vi "Servo MSMT get DPD Config.vi"(8 "error in (no error)":errorcluster, 11 "Servo MSMT in":refnum<class "Servo MSMT.lvclass">) -> (0 "error out":errorcluster, 1 "USE LUT?":bool, 2 "DPD Enabled?":bool, 3 "Servo MSMT out":refnum<class "Servo MSMT.lvclass">, 4 "LUT":string)   [LabVIEW 2018, in "Servo MSMT.lvlib" / "Servo MSMT.lvclass"]
uses:
  Servo MSMT.lvclass
  Plugins/String Database.lvlibp/String Database.lvclass
  Plugins/Test Group Manager.lvlibp/Test Group Manager.lvclass
  Plugins/Test Group Manager.lvlibp/Includes/Test Group/Test Group.lvclass
  <vilib>/ErrorRing/Error Ring.xnode
  <vilib>/Utility/error.llb/Error Cluster From Error Code.vi
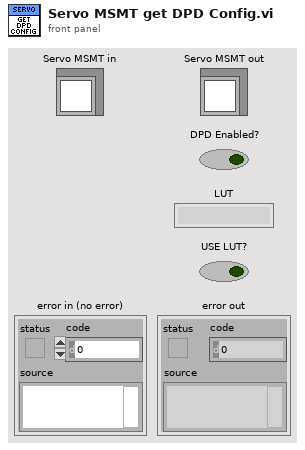
[diagram p1: front panel]
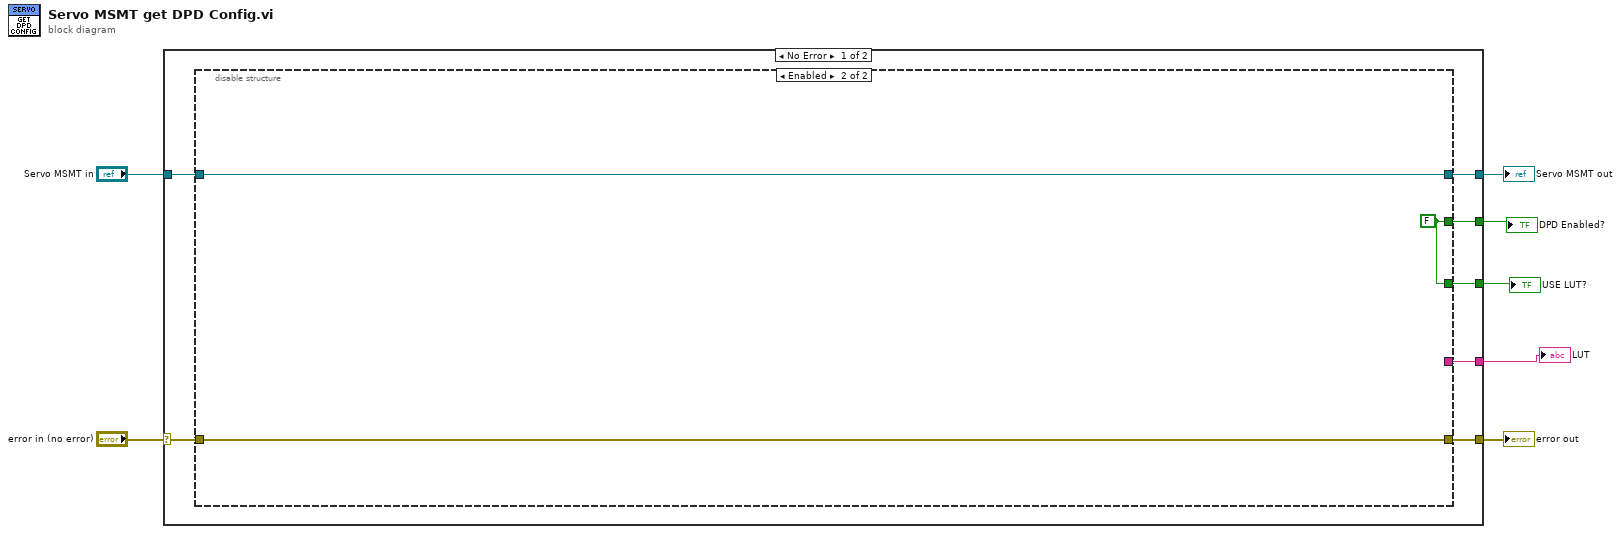
[diagram p0: block diagram]
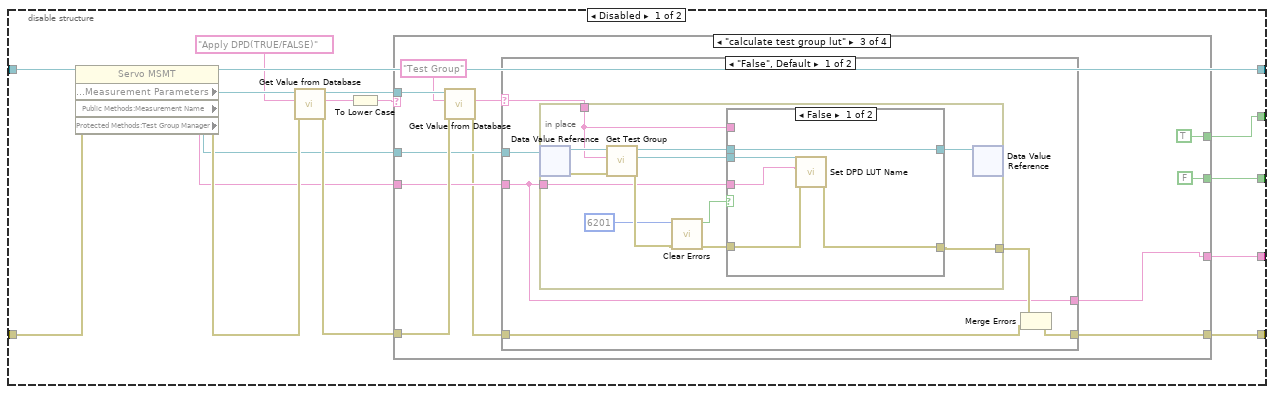
[diagram p2: hidden frame]
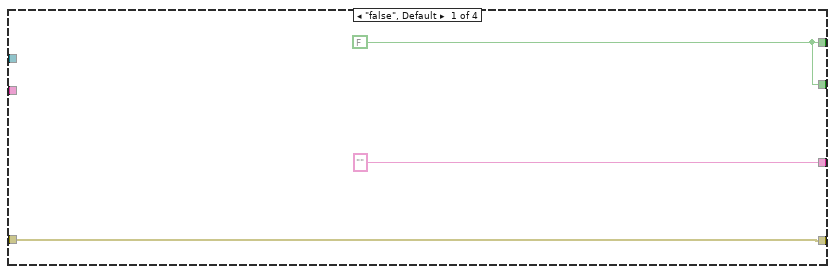
[diagram p3: hidden frame]
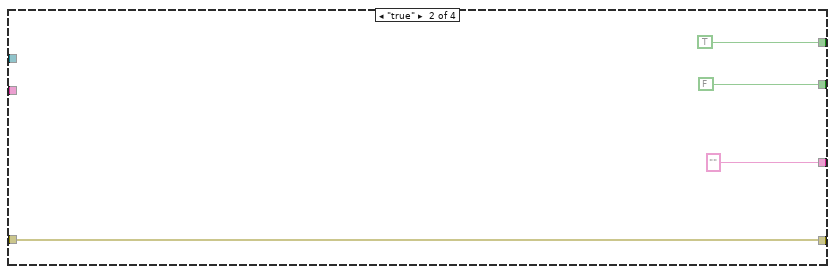
[diagram p4: hidden frame]
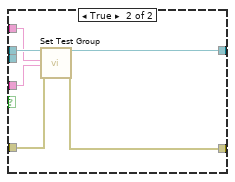
[diagram p5: hidden frame]
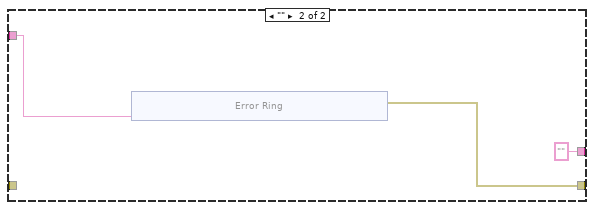
[diagram p6: hidden frame]
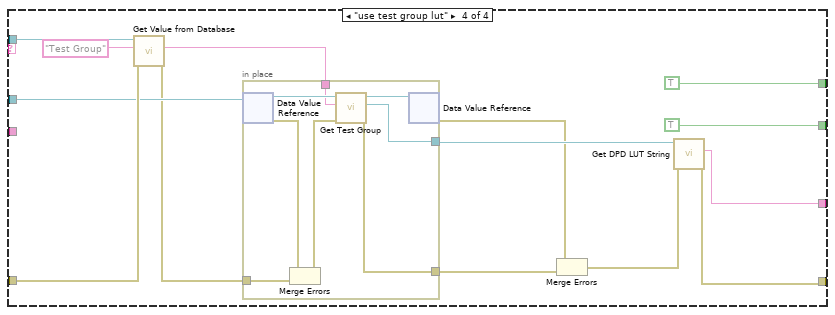
[diagram p7: hidden frame]
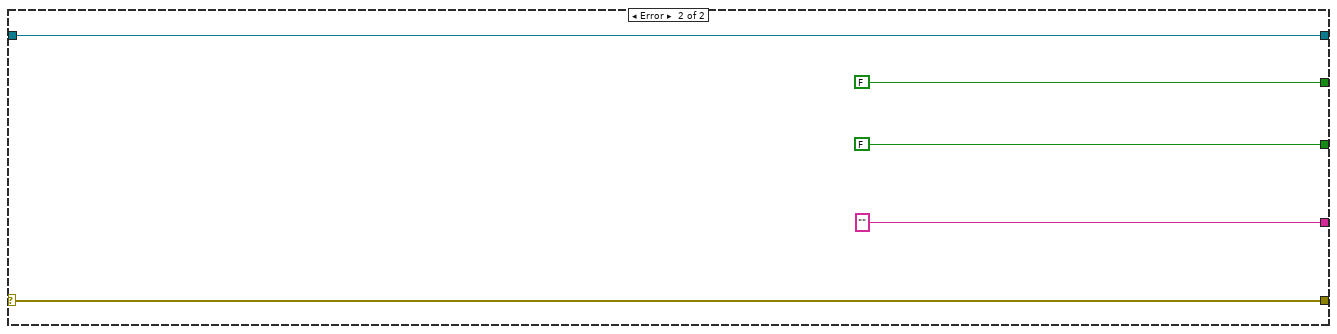
[diagram p8: hidden frame]
diagram:
  n1 = case shown="No Error" "error in (no error)" {
    selector: "error in (no error)" -> [w14 w117]
    tunnel: [w9 w117] -> w6
    tunnel: [w12 w116] -> w4
    tunnel: "Servo MSMT in" -> [w13 w116]
    tunnel: [w11 FALSE] -> w3
    tunnel: [w10 FALSE] -> w2
    tunnel: [w8 "" ("Entry Value")] -> w1
    frame No Error {
      n2 = disable-structure shown="Enabled" {
        disable-tunnel: w14 -> [w30 w111]
        disable-tunnel: w13 -> [w29 w112]
        disable-tunnel: [w28 w112] -> w12
        disable-tunnel: [w22 w110] -> w11
        disable-tunnel: [w21 w110] -> w10
        disable-tunnel: [w20 w111] -> w9
        disable-tunnel: [w18 _] -> w8
        frame Disabled {
          n3 = property class="Servo MSMT"(reference=w29, error in=w30) -> (reference out=w28:refnum<class "Servo MSMT.lvclass">, error out=w26:errorcluster, "Protected Methods:Measurement Parameters"=w27:refnum<class "String Database.lvclass">, "Public Methods:Measurement Name"=w15:string, "Protected Methods:Test Group Manager"=w16:refnum<data-value>)
          n4 = call "Get Value from Database.vi"("error in (no error)"=w26, "Entry Name"="Apply DPD(TRUE/FALSE)", "Message in"=w27) -> ("error out"=w19:errorcluster, "Entry Value"=w24:string, "Message out"=w23:refnum<class "String Database.lvclass">)  [unwired: 5 in, 1 out]
          n5 = To Lower Case(string=w24) -> (all lower case string=w17:string)
          n6 = case shown="\"calculate test group lut\"" w17 {
            tunnel: w23 -> [_ _ w46 w99]
            tunnel: [w33 TRUE TRUE TRUE] -> w22
            tunnel: [w33 FALSE FALSE TRUE] -> w21
            tunnel: [w31 w34 w39 w88] -> w20
            tunnel: w19 -> [w31 w34 w43 w98]
            tunnel: ["" "" w38 w93] -> w18
            tunnel: w16 -> [_ _ w42 w96]
            tunnel: w15 -> [_ _ w41 _]
            frame "false", Default {
              w33 = FALSE
            }
            frame "true" {
            }
            frame "calculate test group lut" {
              n7 = call "Get Value from Database.vi"("error in (no error)"=w43, "Entry Name"="Test Group", "Message in"=w46) -> ("error out"=w40:errorcluster, "Entry Value"=w44:string)  [unwired: 5 in, 2 out]
              n8 = case shown="\"False\", Default" w44 {
                selector: w44 -> [w53 _]
                tunnel: w42 -> [w54 _]
                tunnel: w41 -> [w49 w80]
                tunnel: w40 -> [w50 _]
                tunnel: [w52 w79] -> w39
                tunnel: [w49 "" ("Protected Methods:Measurement Name")] -> w38
                frame "False", Default {
                  n9 = in-place {
                    in-place-border: w53 -> [w58]
                    in-place-border: w49 -> [w56]
                    in-place-border: [w55] -> w51
                    n10 = in-place-dvr #1(w54) -> (w66:refnum<class "Test Group Manager.lvclass">, w65:errorcluster)
                    n11 = call "Get Test Group.vi"("error in (no error)"=w65, "Test Group Name"=w58, "Test Group Manager in"=w66) -> ("error out"=w64:errorcluster, "Test Group In"=w60:refnum<data-value>, "Test Group Manager out"=w59:refnum<class "Test Group Manager.lvclass">)  [unwired: 6 in]
                    n12 = call <vilib>:"Clear Errors.vi"("error in (no error)"=w64, "specific error code to clear (0: all)"=6201) -> ("error out"=w61:errorcluster, "specific error cleared?"=w62:bool)  [unwired: 4 in]
                    n13 = case shown="False" w62 {
                      tunnel: w61 -> [w69 w77]
                      tunnel: w60 -> [w70 _]
                      tunnel: w59 -> [w71 w76]
                      tunnel: w58 -> [_ w75]
                      tunnel: [w71 w74] -> w57
                      tunnel: w56 -> [w67 w73]
                      tunnel: [w68 w72] -> w55
                      frame False {
                        n14 = call "Set DPD LUT Name.vi"("error in (no error)"=w69, "DPD LUT Name"=w67, "Test Group In"=w70) -> ("error out"=w68:errorcluster)  [unwired: 7 in, 1 out]
                      }
                      frame True {
                        n15 = call "Set Test Group.vi"("Test Group Manager in"=w76, "Test Group Name"=w75, "DPD LUT Name"=w73, "error in (no error)"=w77) -> ("Test Group Manager out"=w74:refnum<class "Test Group Manager.lvclass">, "error out"=w72:errorcluster)  [unwired: 14 in]
                      }
                    }
                    n16 = in-place-dvr #1(w57) -> ()  [unwired: 2 out]
                  }
                  n17 = Merge Errors(w51, w50) -> (w52:errorcluster)
                }
                frame "" {
                  n18 = xnode "Error Ring"("parameter 0"=w80) -> ("error out"=w79:errorcluster)
                }
              }
            }
            frame "use test group lut" {
              n19 = call "Get Value from Database.vi"("error in (no error)"=w98, "Entry Name"="Test Group", "Message in"=w99) -> ("error out"=w92:errorcluster, "Entry Value"=w95:string)  [unwired: 5 in, 2 out]
              n20 = in-place {
                in-place-border: w95 -> [w108]
                in-place-border: [w106] -> w94
                in-place-border: w92 -> [w105]
                in-place-border: [w102] -> w91
                n21 = in-place-dvr #2(w96) -> (w109:refnum<class "Test Group Manager.lvclass">, w104:errorcluster)
                n22 = Merge Errors(w104, w105) -> (w103:errorcluster)
                n23 = call "Get Test Group.vi"("error in (no error)"=w103, "Test Group Name"=w108, "Test Group Manager in"=w109) -> ("error out"=w102:errorcluster, "Test Group In"=w106:refnum<data-value>, "Test Group Manager out"=w107:refnum<class "Test Group Manager.lvclass">)  [unwired: 6 in]
                n24 = in-place-dvr #2(w107) -> (w90:errorcluster)  [unwired: 1 out]
              }
              n25 = Merge Errors(w90, w91) -> (w89:errorcluster)
              n26 = call "Get DPD LUT String.vi"("error in (no error)"=w89, "Test Group In"=w94) -> ("error out"=w88:errorcluster, "DPD LUT"=w93:string)  [unwired: 7 in, 1 out]
            }
          }
        }
        frame Enabled {
          w110 = FALSE
        }
      }
    }
    frame Error {
    }
  }
  "error out" <- w6
  "Servo MSMT out" <- w4
  "DPD Enabled?" <- w3
  "USE LUT?" <- w2
  "LUT" <- w1
